vi "Update Configuration (internal).vi"(11 "configuration":T1) -> ()   [LabVIEW 2020, in "Rename As Application UI.lvlib" / "Configuration.lvlib"]
doc: "This private VI is used where a module updates its own data internally as an atomic bulk operation.\n_____\nBased on DCFG Project Template 1.0.0.21.\n____\nPeloton Config 1.0.0.2\nCopyright (c) 2022, Peloton"
uses:
  Configuration.lvlib
  Configuration--cluster.ctl
  Configuration DVR Global.vi
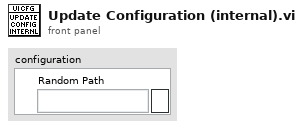
[diagram p1: front panel]
types:
  T1 = typedef "Rename As Application UI.lvlib/Configuration.lvlib/Configuration--cluster.ctl" = cluster{"Random Path":path}
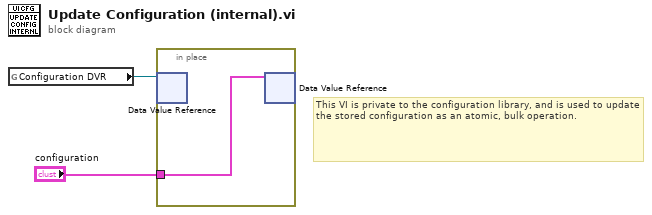
[diagram p0: block diagram]
diagram:
  # "This VI is private to the configuration library, and is used to update the stored configuration as an atomic, bulk operation."
  n1 = global read "Configuration DVR Global.vi" "Configuration DVR"() -> (w2:refnum<data-value>)
  n2 = in-place {
    in-place-border: "configuration" -> [w3]
    n3 = in-place-dvr #1(w2) -> ()  [unwired: 2 out]
    n4 = in-place-dvr #1(w3) -> ()  [unwired: 2 out]
  }
